vi "plcm3CloseUnit.vi"(8 "error in (no error)":errorcluster, 11 "handle in":i16) -> (0 "error out":errorcluster, 3 "handle out":i16)   [LabVIEW 2009]
doc: "This closes the device and should be called before exiting an application."
uses:
  plcm3.dll
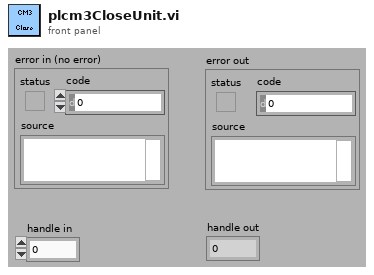
[diagram p1: front panel]
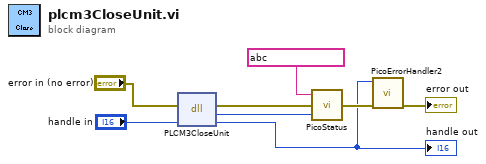
[diagram p0: block diagram]
diagram:
  n1 = dll-call lib="plcm3.dll" fn="PLCM3CloseUnit"(error in="error in (no error)", "handle"="handle in") -> (error out=w5:errorcluster, "Status"=w4:u32, "handle"=w3:i16)  [unwired: 2 in, 1 out]
  "handle out" <- w3
  n2 = call "PicoStatus.vi"("PICO STATUS"=w4, "error in"=w5, "source"=string ?) -> ("error out"=w8:errorcluster)
  n3 = call "PicoErrorHandler2.vi"("error in (no error)"=w8, "handle In"=w3) -> ("error out"=→"error out":errorcluster)  [unwired: 9 in]
